vi "GUID Int to String.vi"(11 "GUID":T1 {"Lo" format="%.0x"; "Hi" format="%.0x"}) -> (3 "uuid":string)   [LabVIEW 2023, in "CEF.lvlib" / "CEF_serializable configuration.lvclass"]
doc: "Copyright 2017 National Instruments Corporation\n\nLicensed under the Apache License, Version 2.0 (the \"License\"); you may not use this file except in compliance with the License. You may obtain a copy of the License at http://www.apache.org/licenses/LICENSE-2.0\nUnless required by applicable law or agreed to in writing, software distributed under the License is distributed on an \"AS IS\" BASIS, WITHOUT WARRANTIES OR CONDITIONS OF ANY KIND, either express or implied. See the License for the specific language governing permissions and limitations under the License."
uses:
  CEF_serializable configuration.lvclass
  Numeric GUID.ctl
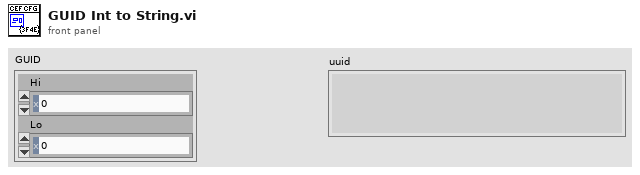
[diagram p1: front panel]
types:
  T1 = typedef "CEF.lvlib/CEF_serializable configuration.lvclass/Numeric GUID.ctl" = cluster{"Hi":u64, "Lo":u64}
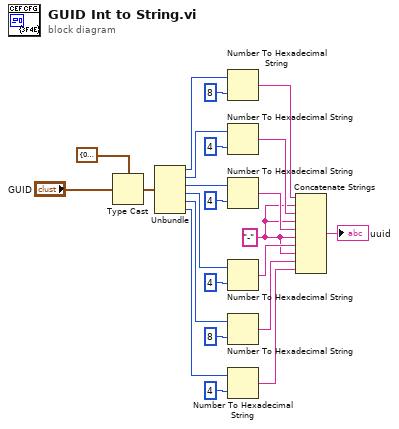
[diagram p0: block diagram]
diagram:
  w10 = "-" ("new element/subarray")
  n1 = Type Cast(type=cluster{u32, u16, u16, u16, u32, u16} {0, 0, 0, 0, 0, 0}, x="GUID") -> (*(type *) &x=w21:cluster{u32, u16, u16, u16, u32, u16})
  n2 = Unbundle(w21) -> (w6:u32, w5:u16, w4:u16, w3:u16, w2:u32, w1:u16)
  n3 = Number To Hexadecimal String(1:i16 8 ("width (-)"), 2:w6) -> (0:w14:string)
  n4 = Number To Hexadecimal String(1:i16 4 ("width (-)"), 2:w5) -> (0:w13:string)
  n5 = Number To Hexadecimal String(1:i16 4 ("width (-)"), 2:w4) -> (0:w12:string)
  n6 = Number To Hexadecimal String(1:i16 4 ("width (-)"), 2:w3) -> (0:w11:string)
  n7 = Number To Hexadecimal String(1:i16 8 ("width (-)"), 2:w2) -> (0:w9:string)
  n8 = Number To Hexadecimal String(1:i16 4 ("width (-)"), 2:w1) -> (0:w8:string)
  n9 = Concatenate Strings(w14, w10, w13, w10, w12, w10, w11, w10, w9, w8) -> (→"uuid":string)
